vi "TPG366_get_gauge.vi"(7 "err_in":errorcluster, 10 "maxi_visa":refnum<visa-resource-name>="COM8") -> (0 "err_out":errorcluster, 3 "Gauge Type":string)   [LabVIEW 2019]
panel:
  out "Overall Status":bool=TRUE
  out "Acknowledgement Status":bool=TRUE
  out "maxi_visa 2":refnum<visa-resource-name>="COM8"
  in  "maxi_b2r 2":u32
  in  "maxi_delay 3":u32=100
  in  "maxi_delay 2":u32
  in  "maxi_b2r":u32
  in  "maxi_delay":u32=100
  # "Gauge Type:\n\nTPR/PCR = Pirani Gauge or Pirani Capacitance Gaige\nIKR = Cold Cathode  Gauge 1E-9 or 1E-11\nPKR = Full Range CC Gauge\nPBR = Full Range BA Gauge\nIMR = Pirani/High Pressure Gauge\nCMR/APR = Linear Gauge\nnoSEN = No Sensor\nnoid = No Identifier"
  # "VISA"
  # "DELAY"
  # "BYTE AT PORT"
  # "STATUS"
  # "ERROR"
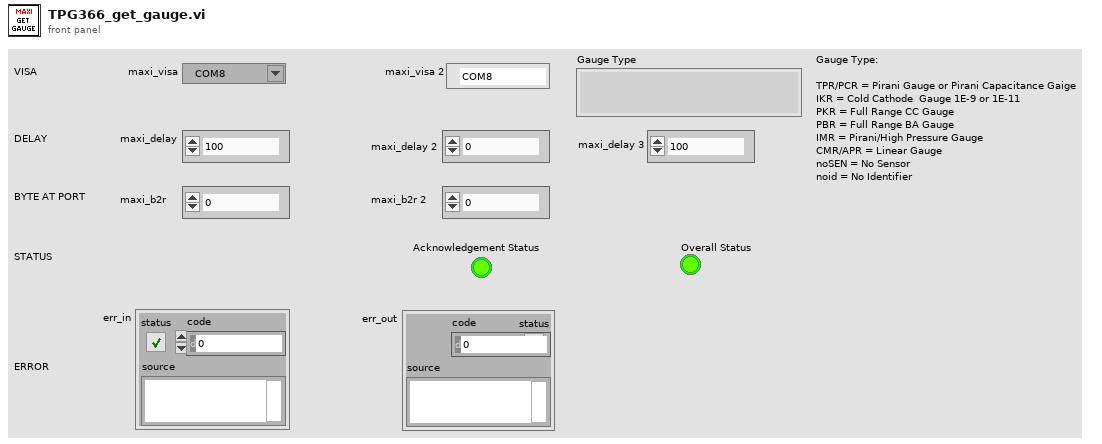
[diagram p1: front panel]
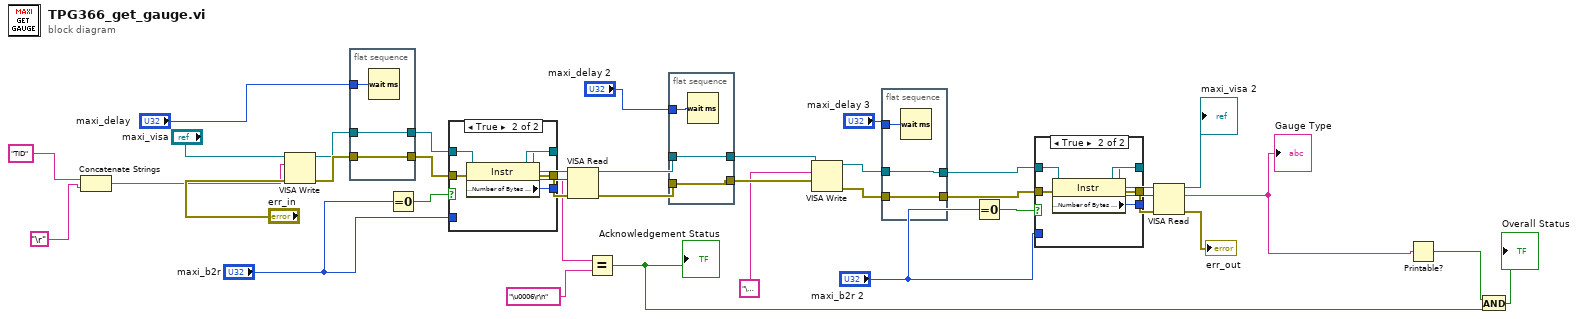
[diagram p0: block diagram]
diagram:
  n1 = Concatenate Strings("TID" ("string"), "\r") -> (w11:string)
  n2 = VISA Write(VISA resource name="maxi_visa", write buffer=w11, error in (no error)="err_in") -> (VISA resource name out=w37:refnum<visa-resource-name>, error out=w39:errorcluster)  [unwired: 1 out]
  n3 = flat-sequence {
    tunnel: w39 -> [w41]
    tunnel: [w41] -> w38
    tunnel: w37 -> [w40]
    tunnel: [w40] -> w36
    tunnel: "maxi_delay" -> [w42]
    frame #0 {
      n4 = Wait (ms)(milliseconds to wait=w42) -> ()  [unwired: 1 out]
    }
  }
  n5 = Equal To 0?(x="maxi_b2r") -> (x = 0?=w32:bool)
  n6 = case shown="True" w32 {
    tunnel: w38 -> [w44 w50]
    tunnel: w36 -> [w45 w49]
    tunnel: [w45 w48] -> w30
    tunnel: [w44 w47] -> w29
    tunnel: [w43 w46] -> w28
    tunnel: "maxi_b2r" -> [w43 _]
    frame False {
    }
    frame True {
      n7 = property class="Instr"(reference=w49, error in=w50) -> (reference out=w48:refnum<visa-resource-name>, error out=w47:errorcluster, "Serial Settings:Number of Bytes at Serial Port"=w46:u32)
    }
  }
  n8 = VISA Read(VISA resource name=w30, byte count=w28, error in (no error)=w29) -> (VISA resource name out=w27:refnum<visa-resource-name>, read buffer=w8:string, error out=w26:errorcluster)  [unwired: 1 out]
  n9 = Equal?(x=w8, y="\u0006\r\n") -> (x = y?=w4:bool)
  "Acknowledgement Status" <- w4
  n10 = flat-sequence {
    tunnel: [w51] -> w24
    tunnel: w27 -> [w53]
    tunnel: [w53] -> w25
    tunnel: "maxi_delay 2" -> [w52]
    tunnel: w26 -> [w51]
    frame #0 {
      n11 = Wait (ms)(milliseconds to wait=w52) -> ()  [unwired: 1 out]
    }
  }
  n12 = VISA Write(VISA resource name=w25, write buffer="\u0005", error in (no error)=w24) -> (VISA resource name out=w17:refnum<visa-resource-name>, error out=w16:errorcluster)  [unwired: 1 out]
  n13 = flat-sequence {
    tunnel: [w55] -> w23
    tunnel: [w56] -> w22
    tunnel: w17 -> [w56]
    tunnel: w16 -> [w55]
    tunnel: "maxi_delay 3" -> [w54]
    frame #0 {
      n14 = Wait (ms)(milliseconds to wait=w54) -> ()  [unwired: 1 out]
    }
  }
  n15 = Equal To 0?(x="maxi_b2r 2") -> (x = 0?=w21:bool)
  n16 = case shown="True" w21 {
    tunnel: w23 -> [w58 w64]
    tunnel: w22 -> [w59 w63]
    tunnel: [w59 w62] -> w20
    tunnel: [w58 w61] -> w19
    tunnel: [w57 w60] -> w18
    tunnel: "maxi_b2r 2" -> [w57 _]
    frame False {
    }
    frame True {
      n17 = property class="Instr"(reference=w63, error in=w64) -> (reference out=w62:refnum<visa-resource-name>, error out=w61:errorcluster, "Serial Settings:Number of Bytes at Serial Port"=w60:u32)
    }
  }
  n18 = VISA Read(VISA resource name=w20, byte count=w18, error in (no error)=w19) -> (VISA resource name out=→"maxi_visa 2":refnum<visa-resource-name>, read buffer=w2:string, error out=→"err_out":errorcluster)  [unwired: 1 out]
  "Gauge Type" <- w2
  n19 = Printable?(1:w2) -> (0:w1:bool)
  n20 = And(x=w1, y=w4) -> (x .and. y?=→"Overall Status":bool)
